vi "GetClassNameArray.vi"(8 "error in (no error)":errorcluster, 10 "ClassName Cache":refnum<data-value>, 11 "LabVIEW Object in":refnum<class>) -> (0 "error out":errorcluster, 3 "Class (child,parent)":T1[](array[typedef]))   [LabVIEW 2020, in "BlueSerialization.lvlib" / "BlueSerializer.lvclass"]
uses:
  BlueSerializer.lvclass
  ClassNameCacheMap.ctl
  ClassNameObj.ctl
  <vilib>/Utility/LVClass/Get LV Class Default Value By Name.vi
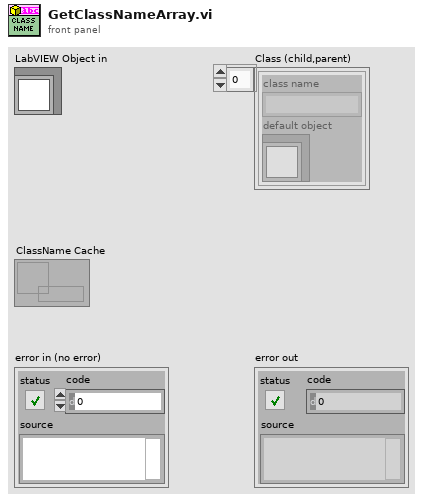
[diagram p1: front panel]
types:
  T1 = typedef "BlueSerialization.lvlib/BlueSerializer.lvclass/ClassNameObj.ctl" = cluster{"class name":string, "default object":refnum<class>}
  T2 = typedef "BlueSerialization.lvlib/BlueSerializer.lvclass/ClassNameCacheMap.ctl" = map{string, T1[]}
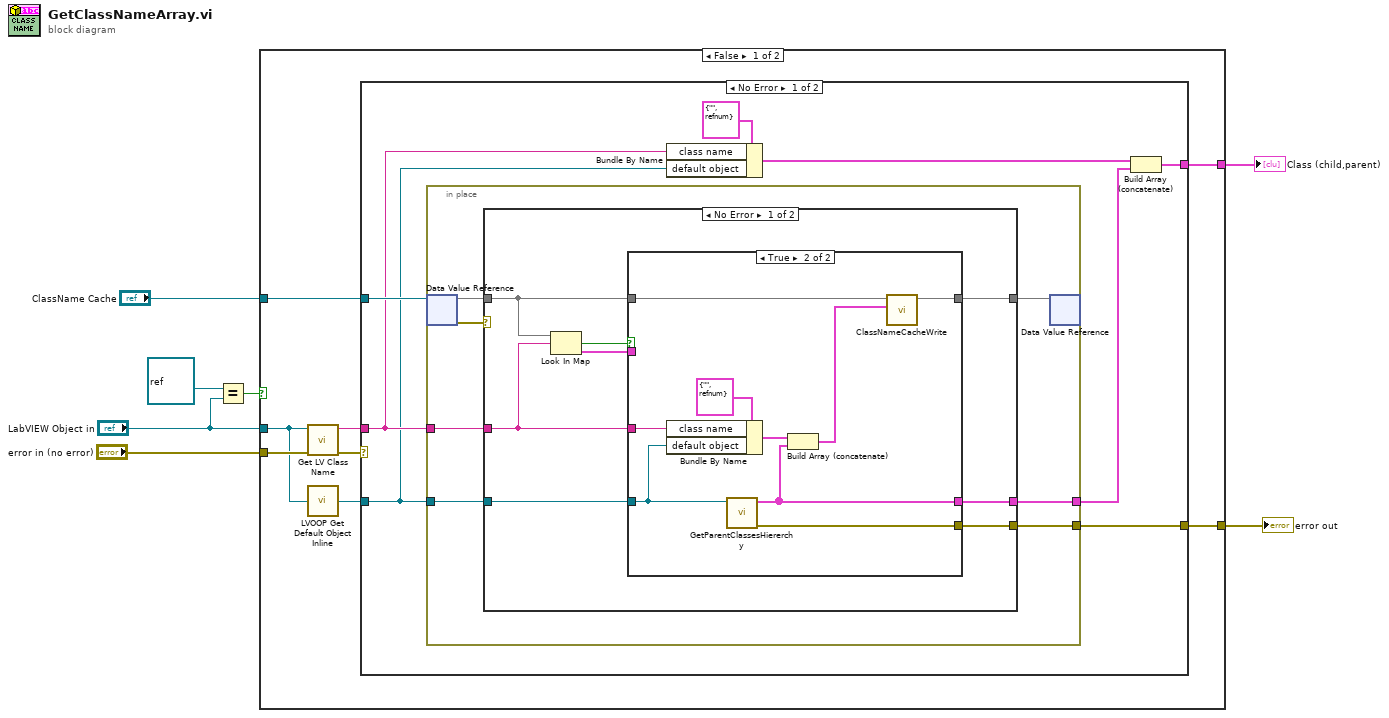
[diagram p0: block diagram]
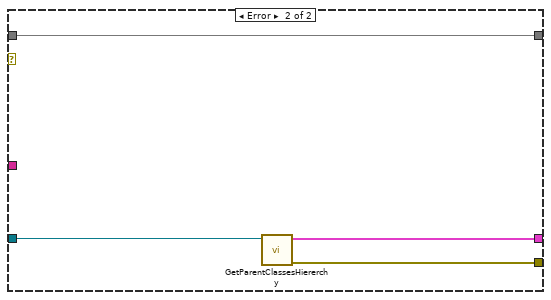
[diagram p3: hidden frame]
diagram:
  n1 = Equal?(x=refnum<class> refnum ("LabVIEW Object"), y="LabVIEW Object in") -> (x = y?=w3:bool)
  n2 = case shown="False" w3 {
    tunnel: "error in (no error)" -> [w14 w55]
    tunnel: [w13 w55] -> w6
    tunnel: [w12 _] -> w1
    tunnel: "LabVIEW Object in" -> [w9 _]
    tunnel: "ClassName Cache" -> [w10 _]
    frame False {
      n3 = call <vilib>:"Get LV Class Name.vi"("error in (no error)"=w14, "object"=w9) -> ("error out"=w11:errorcluster, "class name"=w15:string)  [unwired: 8 in]
      n4 = call "LVOOP Get Default Object Inline.vi"("Object"=w9) -> ("Object Default Instance"=w8:refnum<class>)
      n5 = case shown="No Error" w11 {
        selector: w11 -> [_ w54]
        tunnel: w15 -> [w18 _]
        tunnel: [w20 w54] -> w13
        tunnel: [w22 _] -> w12
        tunnel: w8 -> [w17 _]
        tunnel: w10 -> [w21 _]
        frame No Error {
          n6 = in-place {
            in-place-border: w18 -> [w27]
            in-place-border: [w30] -> w20
            in-place-border: w17 -> [w29]
            in-place-border: [w25] -> w23
            n7 = in-place-dvr #1(w21) -> (w28:T2, w24:errorcluster)
            n8 = case shown="No Error" w24 {
              tunnel: [w38 w52] -> w30
              tunnel: w29 -> [w37 w51]
              tunnel: w28 -> [w35 w53]
              tunnel: w27 -> [w34 _]
              tunnel: [w33 w53] -> w26
              tunnel: [w31 w50] -> w25
              frame No Error {
                n9 = Look In Map(map=w35, key=w34) -> (key not found?=w36:bool, value=w32:T1[])  [unwired: 1 in]
                n10 = case shown="True" w36 {
                  tunnel: [_ w49] -> w38
                  tunnel: w37 -> [_ w43]
                  tunnel: [w39 w41] -> w31
                  tunnel: w35 -> [w40 w48]
                  tunnel: w34 -> [_ w44]
                  tunnel: [w40 w47] -> w33
                  tunnel: w32 -> [w39 _]
                  frame False {
                  }
                  frame True {
                    n11 = Bundle By Name(cluster=T1 {"class name"="", "default object"=refnum} ("Cluster"), "class name"=w44, "default object"=w43) -> (w45:T1)
                    n12 = call "GetParentClassesHiererchy.vi"("LabVIEW Object in"=w43) -> ("error out"=w49:errorcluster, "Class (child,parent)"=w41:T1[])  [unwired: 9 in]
                    n13 = Build Array (concatenate)(w45, w41) -> (w42:T1[])
                    n14 = call "ClassNameCacheWrite.vi"("Class (child,parent)"=w42, "Map"=w48) -> ("Map"=w47:T2)  [unwired: 9 in]
                  }
                }
              }
              frame Error {
                n15 = call "GetParentClassesHiererchy.vi"("LabVIEW Object in"=w51) -> ("error out"=w52:errorcluster, "Class (child,parent)"=w50:T1[])  [unwired: 9 in]
              }
            }
            n16 = in-place-dvr #1(w26) -> ()  [unwired: 2 out]
          }
          n17 = Bundle By Name(cluster=T1 {"class name"="", "default object"=refnum} ("Cluster"), "class name"=w18, "default object"=w17) -> (w16:T1)
          n18 = Build Array (concatenate)(w16, w23) -> (w22:T1[])
        }
        frame Error {
        }
      }
    }
    frame True {
    }
  }
  "error out" <- w6
  "Class (child,parent)" <- w1
